vi "SIRDualStrips.vi"(7 "lower h of strip":dbl format="%.2f", 8 "P":cluster{"x":dbl, "y":dbl, "z":dbl}={"x"=1.0, "y"=-5.0, "z"=1.0} {"x" format="%.2f"; "z" format="%.2f"; "y" format="%.2f"}, 9 "Variables":T1={"sound spd (cm/s)"=150000, "time step (s)"=1e-09} {"time step (s)" format="%.2e"}, 11 "strip":cluster{"Radius":dbl, "h":dbl, "a":dbl}={"Radius"=10.0, "h"=3.0, "a"=5.0} {"Radius" format="%.2f"; "a" format="%.2f"; "h" format="%.2f"}) -> (1 "lower":dbl[](graph), 2 "upper":dbl[](graph), 3 "h out":dbl[](graph), 4 "delay out":i32)   [LabVIEW 2022 SP3]
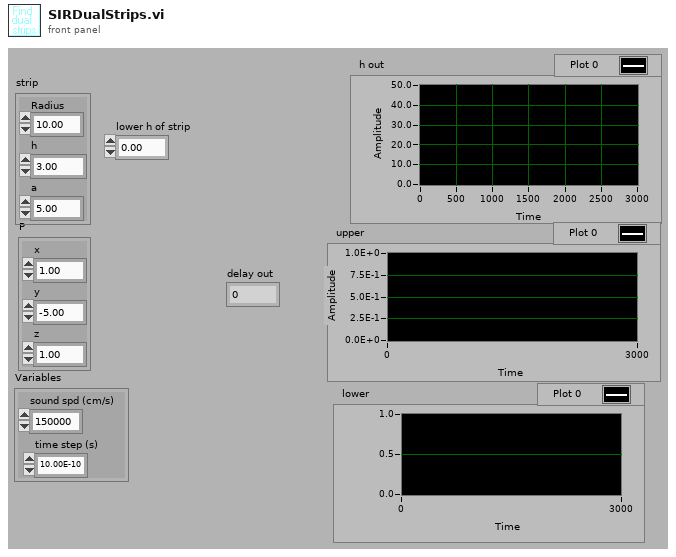
[diagram p1: front panel]
types:
  T1 = cluster{"sound spd (cm/s)":i32, "time step (s)":sgl}
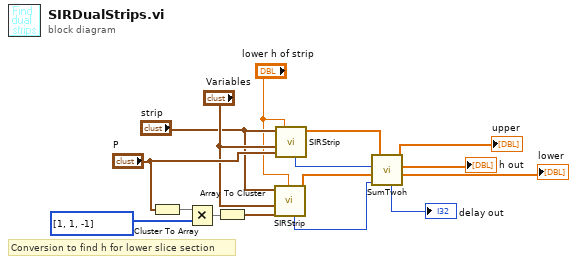
[diagram p0: block diagram]
diagram:
  # "Conversion to find h for lower slice section"
  n1 = Cluster To Array(cluster="P") -> (array=w16:dbl[])
  n2 = Multiply(x=w16, y=i32[] [1, 1, -1] ("Array Constant")) -> (x*y=w14:dbl[])
  n3 = Array To Cluster(array=w14) -> (cluster=w13:cluster{"[0]":dbl, "[1]":dbl, "[2]":dbl})
  n4 = call "SIRStrip.vi"("lower h of strip"="lower h of strip", "P"=w13, "Variables"="Variables", "strip"="strip") -> ("h out"=w1:dbl[], "delay out"=w8:i32)  [unwired: 6 out]
  n5 = call "SIRStrip.vi"("lower h of strip"="lower h of strip", "P"="P", "Variables"="Variables", "strip"="strip") -> ("h out"=w2:dbl[], "delay out"=w9:i32)  [unwired: 6 out]
  n6 = call "SumTwoh.vi"("h1"=w2, "delay1"=w9, "h2"=w1, "delay2"=w8) -> ("delay out"=→"delay out":i32, "upper"=→"upper":dbl[], "h sum"=→"h out":dbl[], "lower"=→"lower":dbl[])  [unwired: 1 out]
